vi "Shared Variable Type Check.vi"(8 "error in (no error)":errorcluster, 10 "Type":T1, 11 "Shared Var in":refnum<k21>) -> (0 "error out":errorcluster, 2 "Matched Type":bool, 3 "Shared Var out":refnum<k21>)   [LabVIEW 2021]
uses:
  <vilib>/Utility/Data Type/Type Definitions/Data Type.ctl
  <vilib>/Utility/error.llb/Error Cluster From Error Code.vi
  <vilib>/ErrorRing/Error Ring.xnode
  <resource>/objmgr/ni.var.rc
  <vilib>/Utility/Data Type/NI_Data Type.lvlib
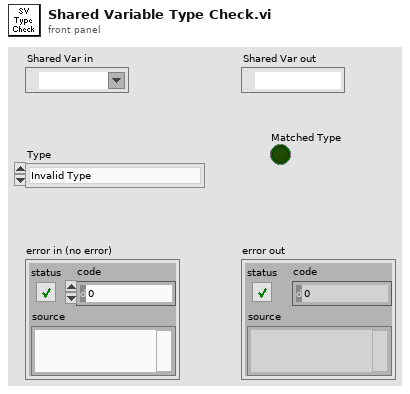
[diagram p1: front panel]
types:
  T1 = typedef "NI_Data Type.lvlib/Data Type.ctl" = enum8{"Invalid Type", "Void", "I8", "I16", "I32", "I64", "U8", "U16", "U32", "U64", "Single Float", "Double Float", "Extended Float", "Single Complex", "Double Complex", "Extended Complex", "Enum U8", "Enum U16", "Enum U32", "Enum U64", "Single Float With Unit", "Double Float With Unit", "Extended Float With Unit", "Single Complex with Unit", "Double Complex with Unit", "Extended Complex with Unit", "Boolean", "String", "Path", "Picture", "Tag", "Array", "Cluster", "Variant", "LV Variant", "Waveform", "Timestamp", "Digital Waveform", "Digital Data", "ExpressData", "Refnum", "External Data", "VI", "Poly VI", "LabVIEW Class Instance", "Fixed Point", "Set Collection", "Map Collection"}
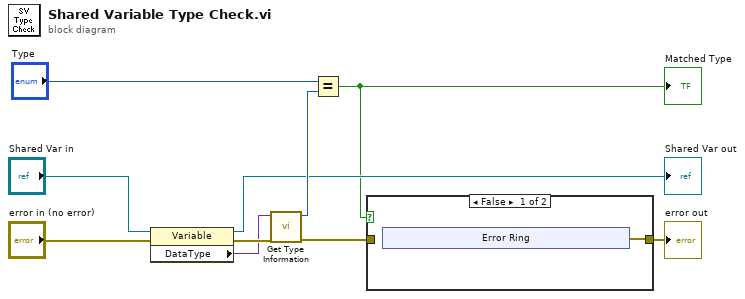
[diagram p0: block diagram]
diagram:
  n1 = property class="Variable"(reference="Shared Var in", error in="error in (no error)") -> (reference out=→"Shared Var out":refnum<k21>, error out=w7:errorcluster, "DataType"=w6:variant)
  n2 = call <vilib>:"Get Type Information.vi"("error in (no error)"=w7, "variant"=w6) -> ("error out"=w3:errorcluster, "type"=w9:T1)  [unwired: 5 in, 3 out]
  n3 = Equal?(x="Type", y=w9) -> (x = y?=w1:bool)
  "Matched Type" <- w1
  n4 = case shown="False" w1 {
    tunnel: w3 -> [_ w16]
    tunnel: [w11 w16] -> w2
    frame False {
      n5 = xnode "Error Ring"() -> ("error out"=w11:errorcluster)
    }
    frame True {
    }
  }
  "error out" <- w2
